vi "CI_IMAQ_Grab.vi"(8 "Camera data":variant, 9 "TrackingParameters":T1={"Corner-based bead pos (out)"=[], "QTrk Instance"={"QTrk Pointer"=0}, "Tracking Config"={"Number of steps"=0, "ZLUT stepsize (um)"=0.0, "Z correction factor"=0.0, "Start piezo Z (um)"=0.0, "Pixel size (nm)"=0.0, "2D Localization Type"=enum."Quadrant Interpolation", "Z Command (None)"=enum."Nothing", "Z Piezo scale"=FALSE}, "ResultManager"={"InstancePtr"=0}, "Send to queue?"=TRUE}, 10 "Output Queue":refnum<queue>, 11 "GrabControlQueue":refnum<queue>) -> (0 "Camera (out)":variant)   [LabVIEW 2011]
uses:
  Main/Typedefs/CmdData_NewFrame.ctl
  <vilib>/vision/Image Controls.llb/IMAQ Image.ctl
  Main/Typedefs/CmdEnum_CameraFrameType.ctl
  Main/Camera/CIGrabParams.ctl
  qtrk/QTrk.llb/QTrkInstance.ctl
  Main/Typedefs/TrackingConfigType.ctl
  qtrk/QTrk.llb/QTrkLocalizationType.ctl
  qtrk/QTrk.llb/QTrkZCommandType.ctl
  qtrk/QTrk.llb/ResultManagerInstance.ctl
  Main/Camera/CIGrabControlMsg.ctl
  Main/Camera/CIGrabControlMsgEnum.ctl
  GenericIMAQCameraInstance.ctl
  Main/Camera/GenericCameraConfigType.ctl
  qtrk/QTrk.llb/QTrkDLL.vi
panel:
  in  "Update lost frames":bool
  out "Status Information : Lost Frames":u32
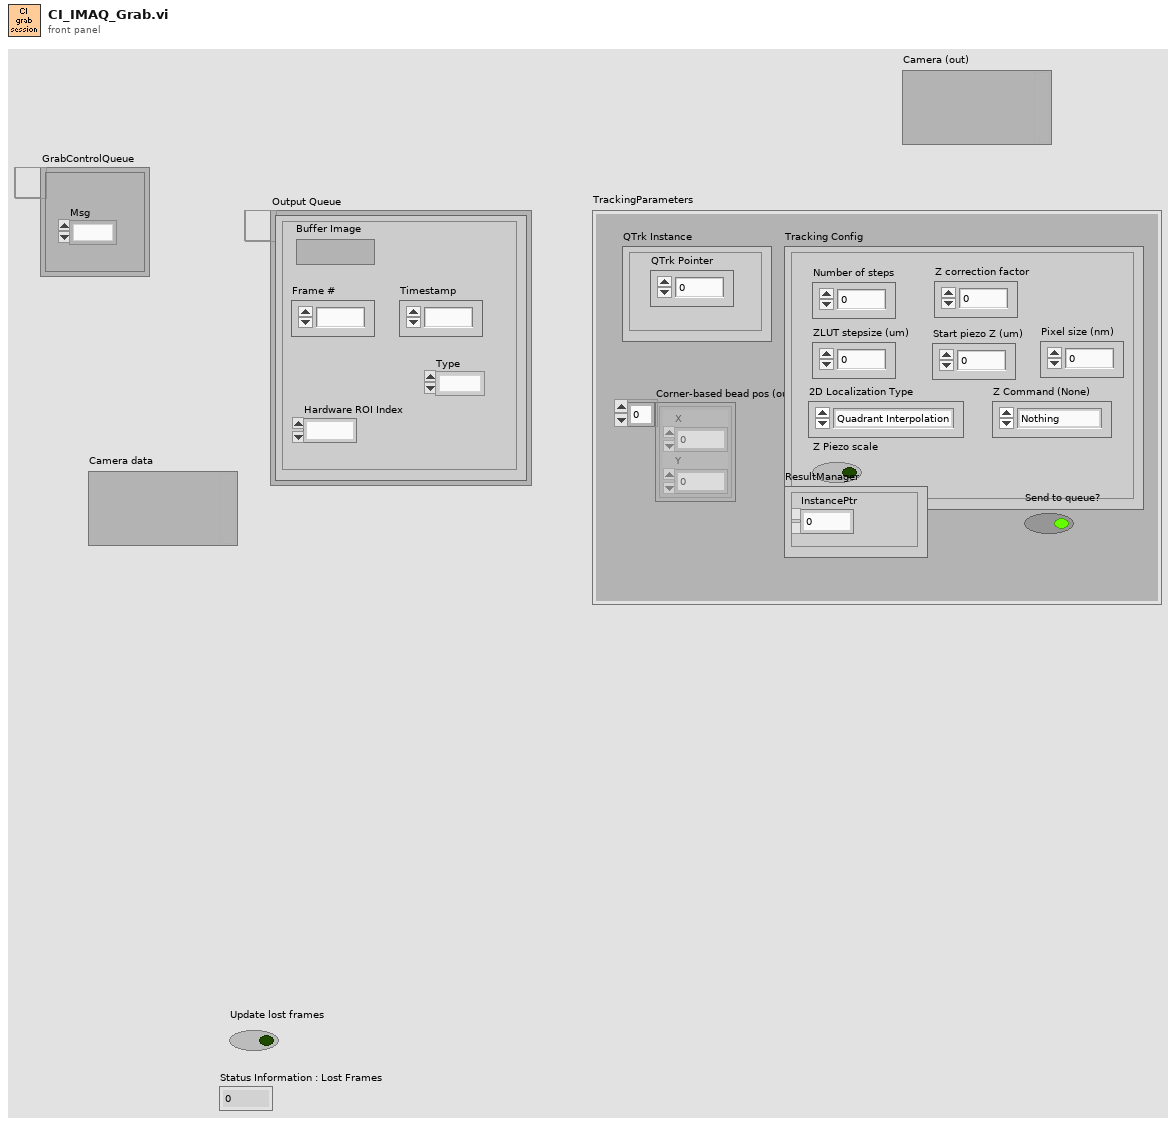
[diagram p1: front panel]
types:
  T1 = typedef "CIGrabParams.ctl" = cluster{"Corner-based bead pos (out)":cluster{"X":i32, "Y":i32}[], "QTrk Instance":T2, "Tracking Config":T3, "ResultManager":T6, "Send to queue?":bool}
  T2 = typedef "QTrkInstance.ctl" = cluster{"QTrk Pointer":u64}
  T3 = typedef "TrackingConfigType.ctl" = cluster{"Number of steps":i32, "ZLUT stepsize (um)":sgl, "Z correction factor":sgl, "Start piezo Z (um)":sgl, "Pixel size (nm)":sgl, "2D Localization Type":T4, "Z Command (None)":T5, "Z Piezo scale":bool}
  T4 = typedef "QTrkLocalizationType.ctl" = enum16{"Center-of-Mass", "1D Cross-Correlation", "Quadrant Interpolation", "Gaussian 2D MLE", "QI + ZLUTAlign", "ZLUTAlign"}
  T5 = typedef "QTrkZCommandType.ctl" = enum16{"Nothing", "ComputeZ", "BuildRadialZLUT", "BuildImageZLUT", "RadialZLUT+ImageZLUT"}
  T6 = typedef "ResultManagerInstance.ctl" = cluster{"InstancePtr":u64}
  T7 = typedef "GenericIMAQCameraInstance.ctl" = cluster{"Session":refnum<k11>, "Settings":T8}
  T8 = typedef "GenericCameraConfigType.ctl" = cluster{"Framerate (Hz)":i32, "Exposure time (us)":i32, "Image size":cluster{"Width":i32, "Height":i32}, "Number of buffers":i32}
  T9 = typedef "CmdEnum_CameraFrameType.ctl" = enum16{"Full", "HardwareROI", "EndGrabMarker"}
  T10 = typedef "CmdData_NewFrame.ctl" = cluster{"Buffer Image":T11, "Frame #":i32, "Hardware ROI Index":i32, "Timestamp":dbl, "Type":T9}
  T11 = typedef "IMAQ Image.ctl" = refnum<image>
  T12 = typedef "CIGrabControlMsg.ctl" = cluster{"Msg":T13}
  T13 = typedef "CIGrabControlMsgEnum.ctl" = enum16{"Stop", "EnableTracking", "DisableTracking"}
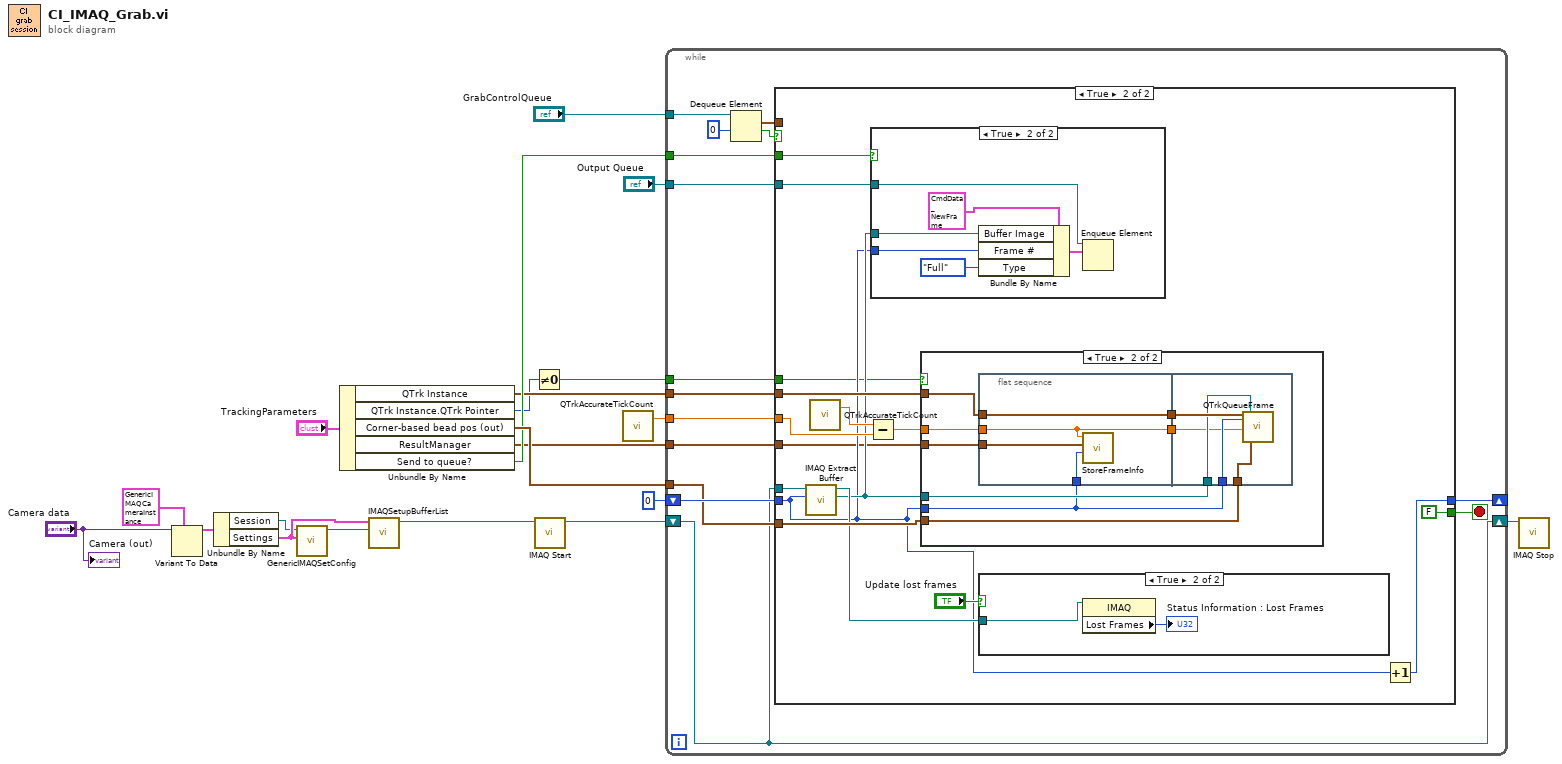
[diagram p0: block diagram]
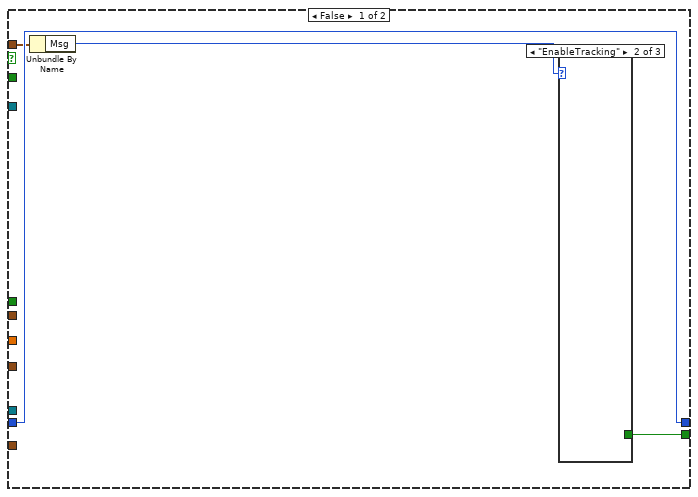
[diagram p2: hidden frame]
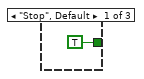
[diagram p3: hidden frame]
diagram:
  n1 = Variant To Data(type=T7 {"Session"=refnum, "Settings"={"Framerate (Hz)"=1, "Exposure time (us)"=50, "Image size"={"Width"=1280, "Height"=1024}, "Number of buffers"=0}} ("Camera data"), Variant="Camera data") -> (data=w17:T7)  [unwired: 1 in, 1 out]
  n2 = Unbundle By Name(w17) -> ("Session"=w2:refnum<k11>, "Settings"=w3:T8)
  n3 = call "GenericIMAQSetConfig.vi"("Camera"=w3, "IMAQ Session In"=w2) -> ("IMAQ Session Out"=w1:refnum<k11>)  [unwired: 9 in]
  n4 = Unbundle By Name("TrackingParameters") -> ("QTrk Instance"=w7:T2, "QTrk Instance.QTrk Pointer"=w6:u64, "Corner-based bead pos (out)"=w12:cluster{"X":i32, "Y":i32}[], "ResultManager"=w9:T6, "Send to queue?"=w11:bool)
  n5 = call "IMAQSetupBufferList.vi"("IMAQ Session In"=w1, "Camera"=w3) -> ("IMAQ Refnum out"=w4:refnum<k11>)  [unwired: 9 in]
  n6 = Not Equal To 0?(x=w6) -> (x != 0?=w5:bool)
  n7 = call <vilib>:"IMAQ Start.vi"("IMAQ Session In"=w4) -> ("IMAQ Session Out"=w16:refnum<k11>)  [unwired: 9 in, 1 out]
  n8 = call "QTrkAccurateTickCount.vi"() -> ("tick count (ms)"=w14:dbl)  [unwired: 2 in, 1 out]
  n9 = while {
    tunnel: "GrabControlQueue" -> [w35]
    shift-right: [w31] -> _
    shift-left: 0 ("Frame number") -> [w32]
    shift-right: [w26] -> w15
    shift-left: w16 -> [w26]
    tunnel: w7 -> [w30]
    tunnel: w12 -> [w27]
    tunnel: w14 -> [w29]
    tunnel: w11 -> [w24]
    tunnel: "Output Queue" -> [w23]
    tunnel: w9 -> [w22]
    tunnel: w5 -> [w21]
    stop <- w25 stop-if-true
    n10 = Dequeue Element(queue=w35, timeout in ms (-1)=0) -> (element=w28:T12, timed out?=w33:bool)  [unwired: 1 in, 2 out]
    n11 = case shown="True" w33 {
      tunnel: w32 -> [w39 w46]
      tunnel: [w39 w56] -> w31
      tunnel: w30 -> [_ w55]
      tunnel: w29 -> [_ w54]
      tunnel: w28 -> [w38 _]
      tunnel: [w36 FALSE ("Quit app")] -> w25
      tunnel: w27 -> [_ w51]
      tunnel: w26 -> [_ w50]
      tunnel: w24 -> [_ w41]
      tunnel: w23 -> [_ w45]
      tunnel: w22 -> [_ w42]
      tunnel: w21 -> [_ w43]
      frame False {
        n12 = Unbundle By Name(w38) -> ("Msg"=w37:T13)
        n13 = case shown="\"EnableTracking\"" w37 {
          tunnel: [TRUE ("Quit app") _ _] -> w36
          frame "Stop", Default {
          }
          frame "EnableTracking" {
          }
          frame "DisableTracking" {
          }
        }
      }
      frame True {
        n14 = call <vilib>:"IMAQ Extract Buffer.vi"("Buffer to extract"=w46, "IMAQ Session In"=w50) -> ("Image Out"=w47:T11, "IMAQ Session Out"=w49:refnum<k11>)  [unwired: 4 in, 4 out]
        n15 = call "QTrkAccurateTickCount.vi"() -> ("tick count (ms)"=w53:dbl)  [unwired: 2 in, 1 out]
        n16 = Subtract(x=w53, y=w54) -> (x-y=w44:dbl)
        n17 = case shown="True" w41 {
          tunnel: w47 -> [_ w61]
          tunnel: w46 -> [_ w60]
          tunnel: w45 -> [_ w57]
          frame False {
          }
          frame True {
            n18 = Bundle By Name(cluster=T10 {"Buffer Image"=refnum, "Frame #"=0, "Hardware ROI Index"=0, "Timestamp"=0.0, "Type"=enum."Full"} ("element"), "Buffer Image"=w61, "Frame #"=w60, "Type"=CmdEnum_CameraFrameType."Full") -> (w59:T10)
            n19 = Enqueue Element(queue=w57, element=w59) -> ()  [unwired: 2 in, 3 out]
          }
        }
        n20 = case shown="True" w43 {
          tunnel: w46 -> [_ w65]
          tunnel: w55 -> [_ w72]
          tunnel: w44 -> [_ w69]
          tunnel: w47 -> [_ w71]
          tunnel: w51 -> [_ w70]
          tunnel: w42 -> [_ w66]
          frame False {
          }
          frame True {
            n21 = flat-sequence {
              tunnel: w69 -> [w75]
              tunnel: w72 -> [w76]
              tunnel: [w76] -> w68
              tunnel: [w75] -> w67
              tunnel: w66 -> [w74]
              tunnel: w65 -> [w73]
              tunnel: w65 -> [w80]
              tunnel: w71 -> [w79]
              tunnel: w70 -> [w78]
              tunnel: w68 -> [w81]
              tunnel: w67 -> [w77]
              frame #0 {
                n22 = call "StoreFrameInfo.vi"("frame"=w73, "ResultManager"=w74, "Timestamp"=w75) -> ()  [unwired: 9 in]
              }
              frame #1 {
                n23 = call "QTrkQueueFrame.vi"("QTrk Instance"=w81, "frame#"=w80, "timestamp"=w77, "Image"=w79, "ROI Positions (corner-based)"=w78) -> ()  [unwired: 12 in, 3 out]
              }
            }
          }
        }
        n24 = case shown="True" "Update lost frames" {
          tunnel: w49 -> [_ w64]
          frame False {
          }
          frame True {
            n25 = property class="IMAQ"(reference=w64) -> ("Lost Frames"=→"Status Information : Lost Frames":u32)  [unwired: 1 in, 2 out]
          }
        }
        n26 = Increment(x=w46) -> (x+1=w56:i32)
      }
    }
  }
  n27 = call <vilib>:"IMAQ Stop.vi"("IMAQ Session In"=w15) -> ()  [unwired: 9 in, 2 out]
  "Camera (out)" <- "Camera data"
